vi "CompileSequence.vi"(1 "Sequence":string="Zero(0.02)\nOne(0.02)\nZero(0.02)\nOne(0.02)\nZero(1)\nOne(1)\nZero(1)\nOne(1)\nZero(1)\nOne(1)\n", 2 "Chapter":string="Chapter(DopplerCooling,\n10100000 00000000 00000000)\nChapter(Pump,\n01000000 00000000 00000000)\nChapter(Pulsed,\n00100000 00000000 00000000,\n00000100 00000000 00000000,\n00000000 10000000 00000000,\n01000000 00000000 01000000)\nChapter(Zero,\n00000000 00000000 00000000)\nChapter(One,\n11111111 11111111 11111111)") -> (0 "Compiled Sequence":string)   [LabVIEW 2014]
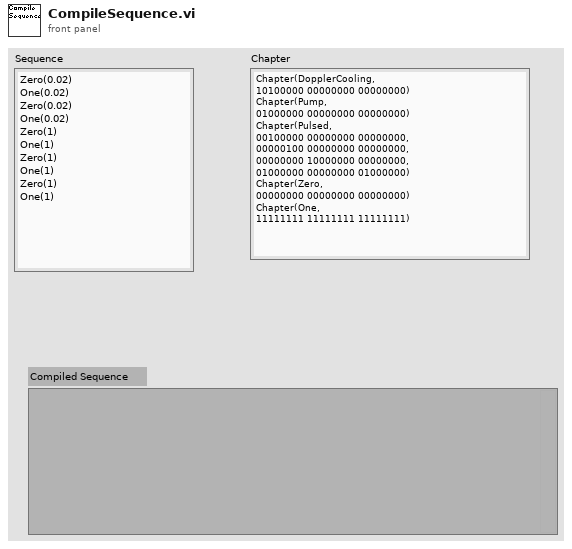
[diagram p1: front panel]
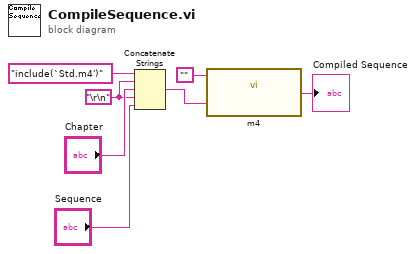
[diagram p0: block diagram]
diagram:
  w1 = "\r\n"
  n1 = Concatenate Strings("include(`Std.m4')", w1, "Chapter", w1, "Sequence") -> (w5:string)
  n2 = call "m4.vi"("input"=w5, "file"="") -> ("output"=→"Compiled Sequence":string)  [unwired: 1 in]
